vi "Main_VI_2.vi"   [LabVIEW 2020]
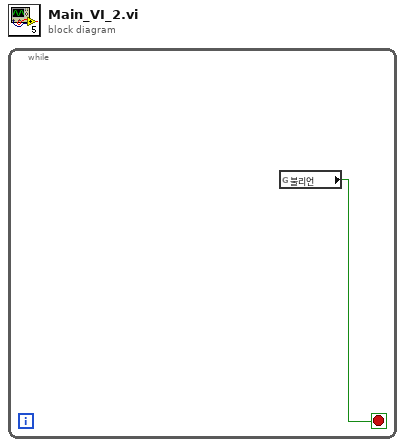
[diagram p0: block diagram]
diagram:
  n1 = while {
    stop <- w1 stop-if-true
    n2 = global read "TEST_글로벌.vi" "불리언"() -> (w1:bool)
  }
